vi "FTW-Example-SLASD-Remove Actor.vi"(0 "FTW-Example-SLASD In":refnum<class "FTW-Example-SLASD.lvclass">, 7 "Actor Address to Remove":string, 11 "error in (no error)":errorcluster) -> (4 "FTW-Example-SLASD Out":refnum<class "FTW-Example-SLASD.lvclass">, 15 "error out":errorcluster)   [LabVIEW 2013, in "FTW-Example-SLASD.lvclass"]
uses:
  FTW-Example-SLASD.lvclass
  Actor/src/Connector/FTW-ActorConnector.lvclass
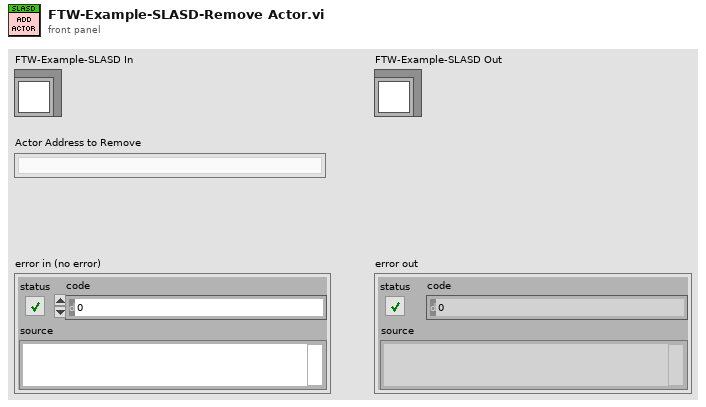
[diagram p1: front panel]
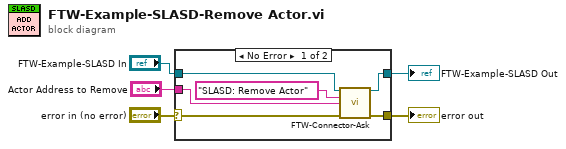
[diagram p0: block diagram]
diagram:
  n1 = case shown="No Error" "error in (no error)" {
    selector: "error in (no error)" -> [w9 w12]
    tunnel: "FTW-Example-SLASD In" -> [w11 w13]
    tunnel: [w10 w13] -> w3
    tunnel: [w8 w12] -> w2
    tunnel: "Actor Address to Remove" -> [w6 _]
    frame No Error {
      n2 = call "FTW-Connector-Ask.vi"("FTW Actor Connector"=w11, "Request Header"="SLASD: Remove Actor", "Request Body"=w6, "error in"=w9) -> ("FTW Actor Connector out"=w10:refnum<class "FTW-Example-SLASD.lvclass">, "error out"=w8:errorcluster)  [unwired: 6 in, 4 out]
    }
    frame Error {
    }
  }
  "FTW-Example-SLASD Out" <- w3
  "error out" <- w2
